vi "Sub_Large_Matrix_Population.vi"(10 "No. of Nodes":i32, 11 "Element Matrix":dbl[][](array[numeric])) -> (3 "Matrix w/o BC":dbl[][](array[numeric]))   [LabVIEW 2021]
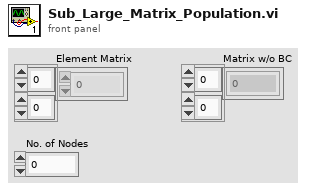
[diagram p1: front panel]
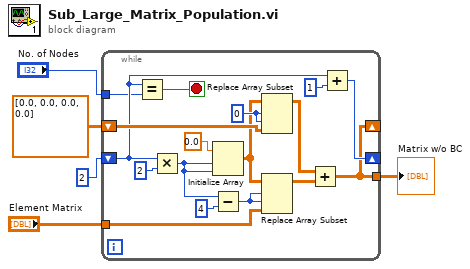
[diagram p0: block diagram]
diagram:
  n1 = while {
    shift-right: [w8] -> _
    shift-left: dbl[][] [[0.0, 0.0], [0.0, 0.0]] -> [w19]
    shift-right: [w15] -> _
    shift-left: 2 -> [w12]
    tunnel: "No. of Nodes" -> [w11]
    tunnel: "Element Matrix" -> [w9]
    tunnel: [w8] -> w4
    stop <- w10 stop-if-true
    w18 = 0 ("index")
    n2 = Equal?(x=w12, y=w11) -> (x = y?=w10:bool)
    n3 = Multiply(x=w12, y=2) -> (x*y=w7:i32)
    n4 = Initialize Array(0.0 ("element"), w7, w7) -> (w6:dbl[][])
    n5 = Subtract(x=w7, y=4) -> (x-y=w17:i32)
    n6 = Replace Array Subset(array=w6, new element=w19, index (row)=w18, index (col)=w18) -> (w14:dbl[][])
    n7 = Replace Array Subset(array=w6, new element=w9, index (row)=w17, index (col)=w17) -> (w13:dbl[][])
    n8 = Add(x=w14, y=w13) -> (x+y=w8:dbl[][])
    n9 = Add(x=w12, y=1) -> (x+y=w15:i32)
  }
  "Matrix w/o BC" <- w4
